vi "Read Roles.vi"(8 "error in (no error)":errorcluster, 11 "DirectKickPlay in":refnum<class "DirectKickPlay.lvclass">) -> (0 "error out":errorcluster, 2 "Roles":T1, 3 "DirectKickPlay out":refnum<class "DirectKickPlay.lvclass">)   [LabVIEW 2023, in "DirectKickPlay.lvclass"]
uses:
  DirectKickPlay.lvclass
  FollowAttackerRole_class/FollowAttackerRole.lvclass
  ShootRole_class/ShootRole.lvclass
  DirectKickPlay.lvclass/DirectKickPlay.ctl
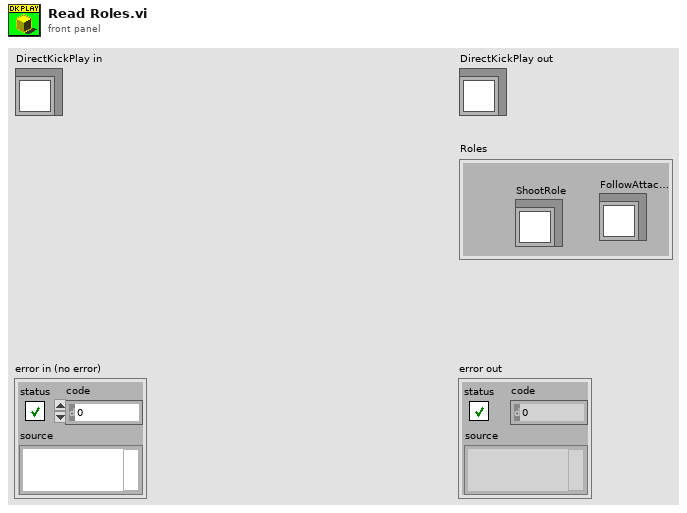
[diagram p1: front panel]
types:
  T1 = cluster{"FollowAttackerRole":refnum<class "FollowAttackerRole.lvclass">, "ShootRole":refnum<class "ShootRole.lvclass">}
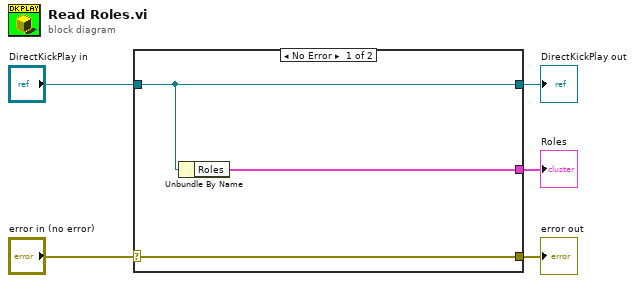
[diagram p0: block diagram]
diagram:
  n1 = case shown="No Error" "error in (no error)" {
    selector: "error in (no error)" -> [w8 w9]
    tunnel: [w8 w9] -> w4
    tunnel: [w7 w10] -> w2
    tunnel: "DirectKickPlay in" -> [w7 w10]
    tunnel: [w6 _] -> w1
    frame No Error {
      n2 = Unbundle By Name(w7) -> ("Roles"=w6:T1)
    }
    frame Error {
    }
  }
  "error out" <- w4
  "DirectKickPlay out" <- w2
  "Roles" <- w1
